vi "DiffDriveSim_Create_Model.vi"(6 "Encoder Counts/Rev":dbl=360.0, 7 "Robot Physical Info":T1={"Mass_LB"=3.0, "Actual TrackWidth Inch"=21.0, "Skid Factor"=1.75} {"Actual TrackWidth Inch" format="%#_13g"}, 8 "Use Custom Drive":bool, 9 "Custom Drive Info":T6={"Motor Type"=enum."Romi BuiltIn", "Num Motors Per Side"=1, "Wheel Diameter Inch"=7.0, "Gear Ratio"=1.0} {"Gear Ratio" format="%#_13g"; "Wheel Diameter Inch" format="%#_13g"}, 10 "KitBot Drive Info":T2, 11 "Initial Robot Position":T8={"TRANSLATION"={"X"=0.0, "Y"=0.0}, "ROTATION"={"VALUE"=0.0, "COS"=1.0, "SIN"=0.0}} {"ROTATION"."SIN" format="%13.4f"; "ROTATION"."COS" format="%13.4f"; "ROTATION"."VALUE" format="%13.4f"; "TRANSLATION"."Y" format="%14.3f"; "TRANSLATION"."X" format="%14.3f"}) -> (2 "Encoder Ft/Count":dbl, 3 "out DiffDriveTrainSim":T11 {"m_Motor"."Jr_KgM2" format="%13.5p"; "m_Motor"."L_H" format="%13.5p"; "m_Motor"."Kt_NMPerAmp" format="%13.5p"; "m_Motor"."KvINV_RadPerSecPerVolt" format="%13.5p"; "m_Motor"."R_Ohms" format="%13.5p"; "m_Motor"."FreeSpeed_RadPerSec" format="%13.5p"; "m_Motor"."FreeCurrent_Amps" format="%13.5p"; "m_Motor"."StallCurrent_Amps" format="%13.5p"; "m_Motor"."StallTorque_NM" format="%13.5p"; "m_Motor"."nominalVoltage_Volts" format="%13.5p"})   [LabVIEW 2019]
uses:
  <vilib>/Rock Robotics/WPI/ThirdParty/JAS_Junk/TrajLib/TypeDef/DIFF_DRIVE_TRAIN_SIM.ctl
  <vilib>/Rock Robotics/WPI/ThirdParty/JAS_Junk/TrajLib/TypeDef/LINEAR_SYSTEM.ctl
  <vilib>/Analysis/Matrix/Datatypes/RealMatrix.ctl
  <vilib>/Rock Robotics/WPI/ThirdParty/JAS_Junk/TrajLib/TypeDef/DCMOTOR.CTL
  <vilib>/Rock Robotics/WPI/ThirdParty/JAS_Junk/TrajLib/TypeDef/POSE2D.ctl
  <vilib>/Rock Robotics/WPI/ThirdParty/JAS_Junk/TrajLib/TypeDef/TRANSLATION2D.ctl
  <vilib>/Rock Robotics/WPI/ThirdParty/JAS_Junk/TrajLib/TypeDef/ROTATION2D.ctl
  DiffDriveSim_CustomDriveIntoType.ctl
  <vilib>/Rock Robotics/WPI/ThirdParty/JAS_Junk/TrajLib/Enum/DCMOTOR_TYPES_ENUM.ctl
  DiffDriveSim_KitBotDriveInfoType.ctl
  <vilib>/Rock Robotics/WPI/ThirdParty/JAS_Junk/TrajLib/Enum/DIFF_DRIVE_ToughBoxMini_MotorChoice_ENUM.ctl
  <vilib>/Rock Robotics/WPI/ThirdParty/JAS_Junk/TrajLib/Enum/DIFF_DRIVE_KitBot_WheelSize_ENUM.ctl
  <vilib>/Rock Robotics/WPI/ThirdParty/JAS_Junk/TrajLib/Enum/DIFF_DRIVE_ToughBoxMini_GearChoice_ENUM.ctl
  DiffDriveSim_PhysRobotInfoType.ctl
  <vilib>/Rock Robotics/WPI/ThirdParty/JAS_Junk/TrajLib/MatBuilder_Create.vi
  <vilib>/Rock Robotics/WPI/ThirdParty/JAS_Junk/TrajLib/Trajectory_Library.lvlib
  <vilib>/Analysis/Matrix/NI_Matrix.lvlib
panel:
  # "<States, 1>"
  # "<Outputs, 1>"
  # "<Inputs, 1>"
  # "<Outputs, 1>"
  # "<States,States>"
  # "<States,Inputs>"
  # "<Outputs,States>"
  # "<Outputs,Inputs>"
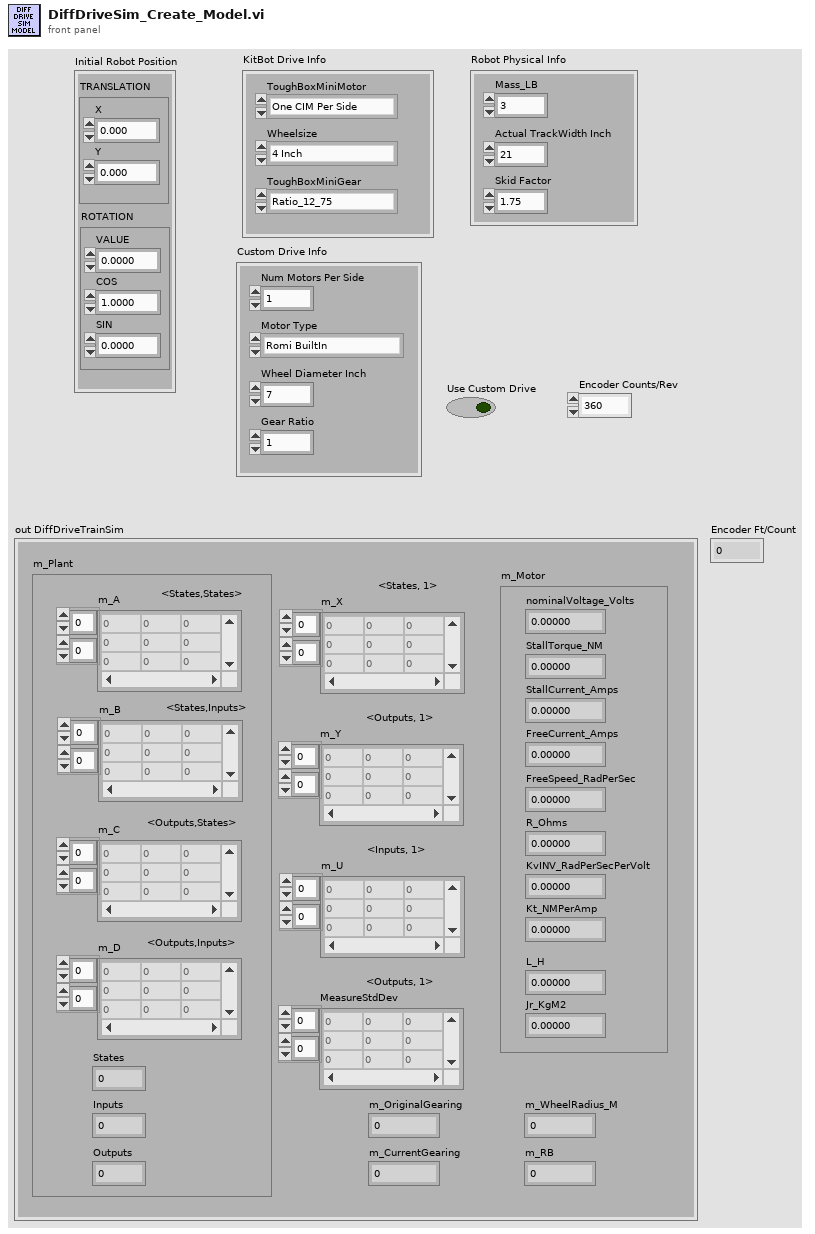
[diagram p1: front panel]
types:
  T1 = typedef "DiffDriveSim_PhysRobotInfoType.ctl" = cluster{"Mass_LB":dbl, "Actual TrackWidth Inch":dbl, "Skid Factor":dbl}
  T2 = typedef "DiffDriveSim_KitBotDriveInfoType.ctl" = cluster{"ToughBoxMiniMotor":T3, "Wheelsize":T4, "ToughBoxMiniGear":T5}
  T3 = typedef "Trajectory_Library.lvlib/DIFF_DRIVE_ToughBoxMini_MotorChoice_ENUM.ctl" = enum16{"One CIM Per Side", "Two CIM Per Side", "One MiniCIM Per Side", "Two Mini CIM Per Side", "Two Falcon Per Side", "Two NEO Per Side"}
  T4 = typedef "Trajectory_Library.lvlib/DIFF_DRIVE_KitBot_WheelSize_ENUM.ctl" = enum16{"4 Inch", "6 Inch", "8 Inch", "10 Inch"}
  T5 = typedef "Trajectory_Library.lvlib/DIFF_DRIVE_ToughBoxMini_GearChoice_ENUM.ctl" = enum16{"Ratio_12_75", "Ratio_10_71", "Ratio_8_45", "Ratio_7_31", "Ratio_5_95"}
  T6 = typedef "DiffDriveSim_CustomDriveIntoType.ctl" = cluster{"Motor Type":T7, "Num Motors Per Side":i32, "Wheel Diameter Inch":dbl, "Gear Ratio":dbl}
  T7 = typedef "Trajectory_Library.lvlib/DCMOTOR_TYPES_ENUM.ctl" = enum16{"CIM", "AndyMark 9015", "Andy Mark RS 775 125", "Bag", "BaneBots RS 550", "BaneBots RS 775", "Falcon 500", "Mini CIM", "NEO", "NEO 550", "Romi BuiltIn", "Vex 775 Pro"}
  T8 = typedef "Trajectory_Library.lvlib/POSE2D.ctl" = cluster{"TRANSLATION":T9, "ROTATION":T10}
  T9 = typedef "Trajectory_Library.lvlib/TRANSLATION2D.ctl" = cluster{"X":dbl, "Y":dbl}
  T10 = typedef "Trajectory_Library.lvlib/ROTATION2D.ctl" = cluster{"VALUE":dbl, "COS":dbl, "SIN":dbl}
  T11 = typedef "Trajectory_Library.lvlib/DIFF_DRIVE_TRAIN_SIM.ctl" = cluster{"m_Plant":T12, "m_X":T13, "m_Y":T13, "m_U":T13, "MeasureStdDev":T13, "m_Motor":T14, "m_OriginalGearing":dbl, "m_CurrentGearing":dbl, "m_WheelRadius_M":dbl, "m_RB":dbl}
  T12 = typedef "Trajectory_Library.lvlib/LINEAR_SYSTEM.ctl" = cluster{"m_A":T13, "m_B":T13, "m_C":T13, "m_D":T13, "States":i32, "Inputs":i32, "Outputs":i32}
  T13 = typedef "NI_Matrix.lvlib/RealMatrix.ctl" = dbl[][]
  T14 = typedef "Trajectory_Library.lvlib/DCMOTOR.CTL" = cluster{"nominalVoltage_Volts":dbl, "StallTorque_NM":dbl, "StallCurrent_Amps":dbl, "FreeCurrent_Amps":dbl, "FreeSpeed_RadPerSec":dbl, "R_Ohms":dbl, "KvINV_RadPerSecPerVolt":dbl, "Kt_NMPerAmp":dbl, "L_H":dbl, "Jr_KgM2":dbl}
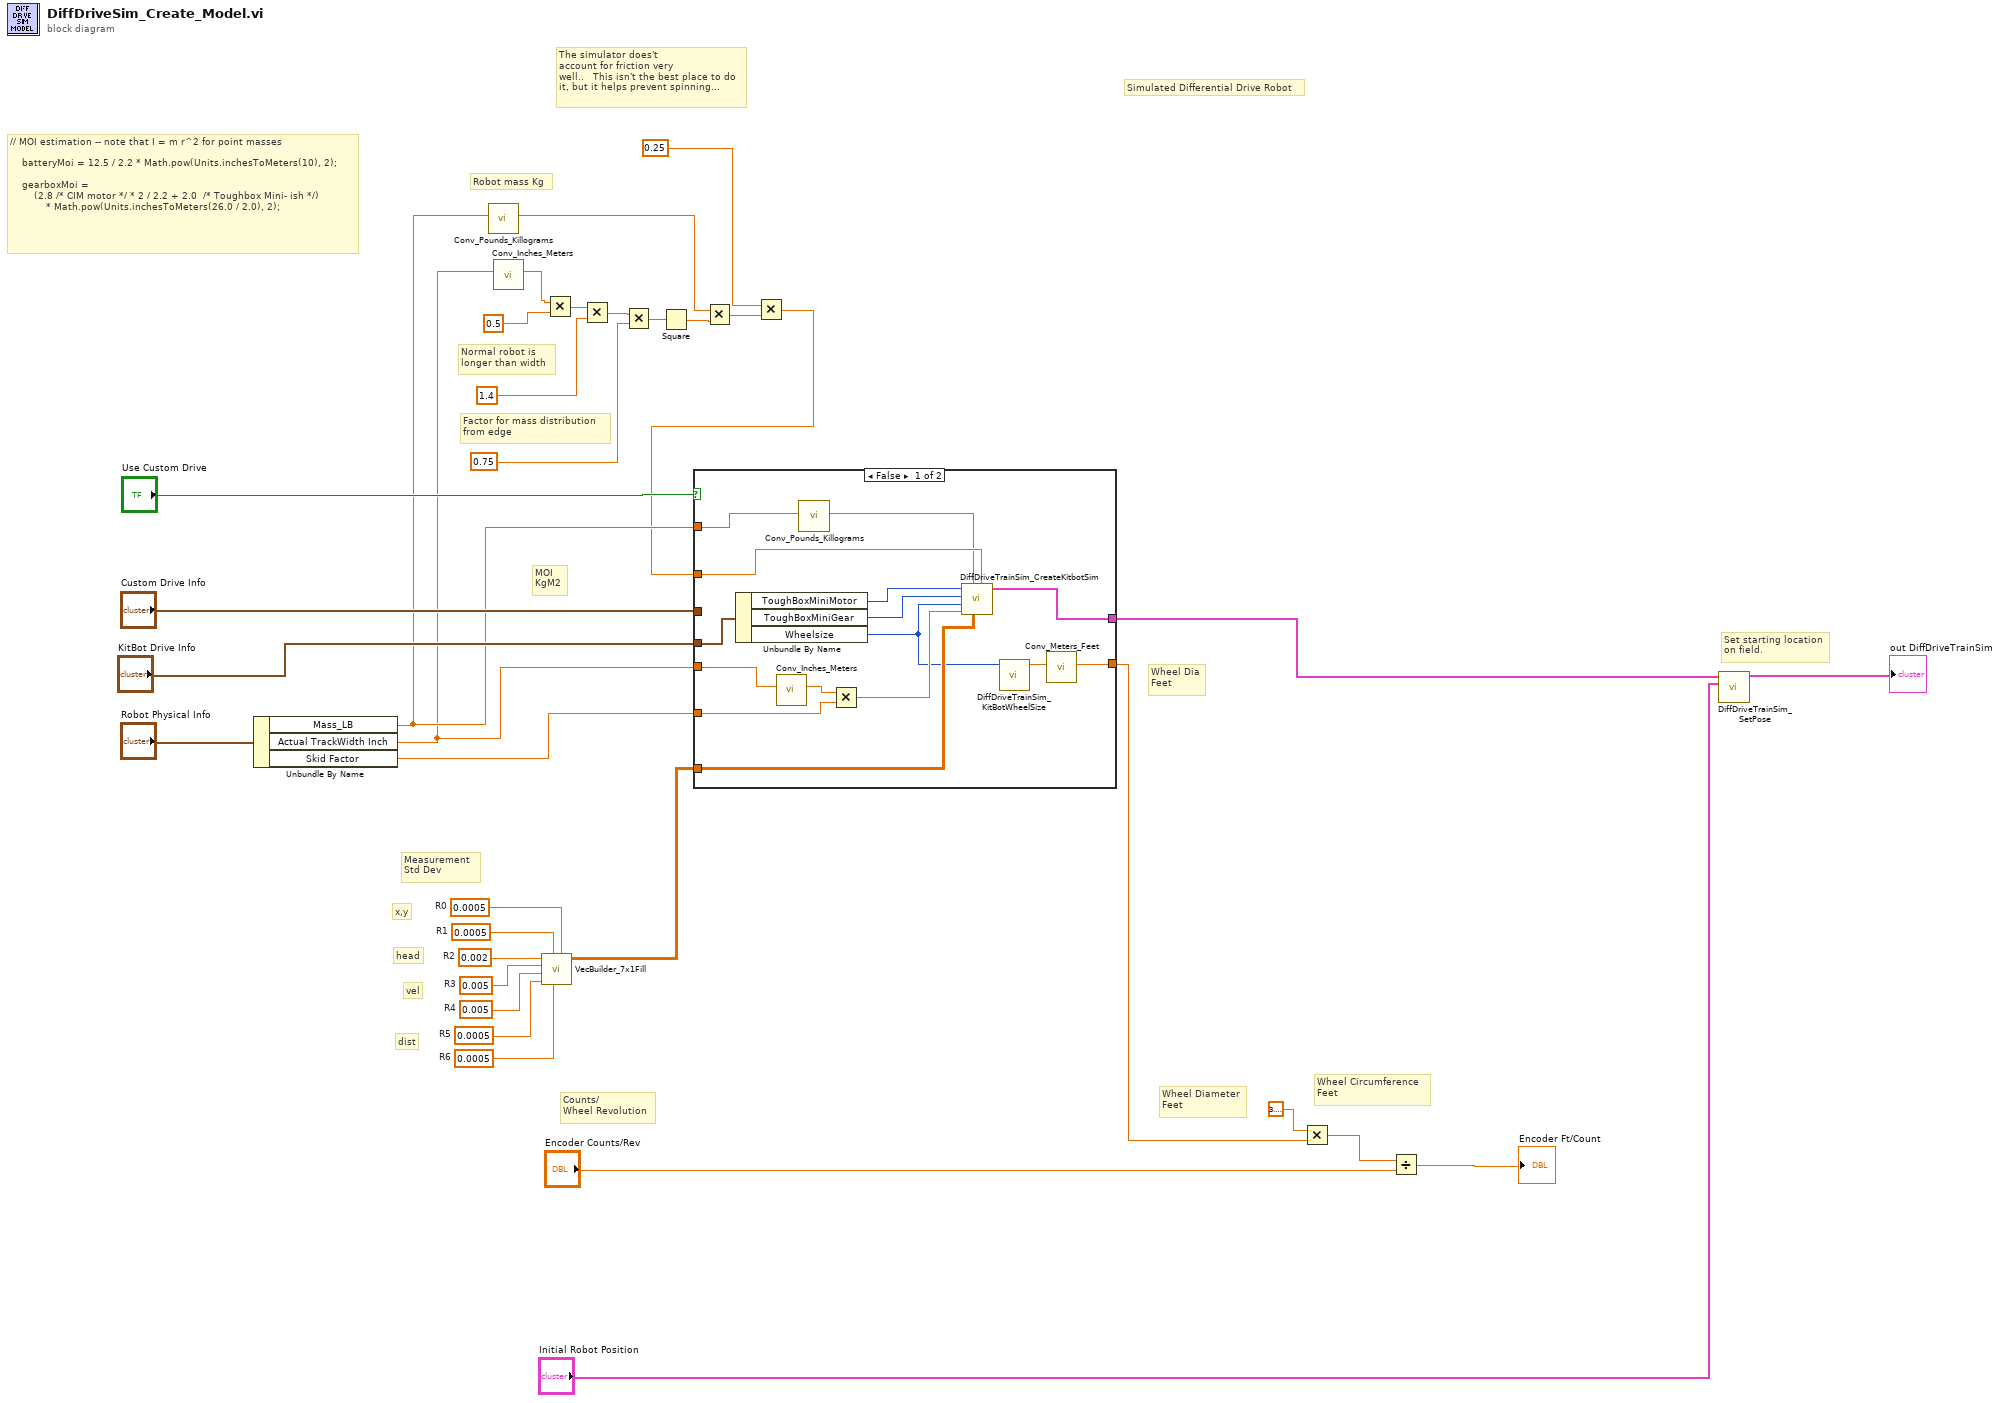
[diagram p0: block diagram]
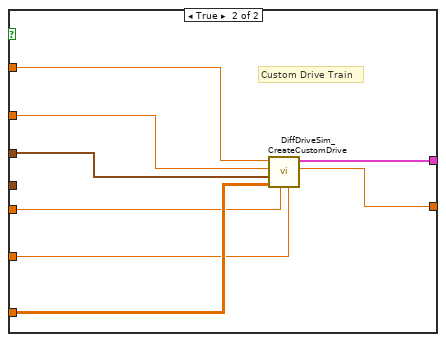
[diagram p2: hidden frame]
diagram:
  w27 = 0.0005  # R6
  w28 = 0.0005  # R5
  w29 = 0.005  # R4
  w30 = 0.005  # R3
  w31 = 0.002  # R2
  w32 = 0.0005  # R1
  w33 = 0.0005  # R0
  # "The simulator does't\naccount for friction very\nwell..   This isn't the best place to do\nit, but it helps prevent spinning..."
  # "Factor for mass distribution \nfrom edge"
  # "Normal robot is\nlonger than width"
  # "Robot mass Kg"
  # "// MOI estimation -- note that I = m r^2 for point masses\n\n    batteryMoi = 12.5 / 2.2 * Math.pow(Units.inchesToMeters(10), 2);\n\n    gearboxMoi =\n        (2.8 /* CIM motor */ * 2 / 2.2 + 2.0 \t/* Toughbox Mini- ish */)\n            * Math.pow(Units.inchesToMeters(26.0 / 2.0), 2);"
  # "Wheel Dia\nFeet"
  # "Wheel Circumference\nFeet"
  # "Wheel Diameter\nFeet"
  # "Counts/\nWheel Revolution"
  # "Set starting location\non field."
  # "Measurement \nStd Dev"
  # "MOI\nKgM2"
  # "dist"
  # "vel"
  # "head"
  # "x,y"
  # "Simulated Differential Drive Robot"
  n1 = Unbundle By Name("Robot Physical Info") -> ("Mass_LB"=w14:dbl, "Actual TrackWidth Inch"=w12:dbl, "Skid Factor"=w15:dbl)
  n2 = call <vilib>:"Conv_Pounds_Killograms.vi"("Pounds"=w14) -> ("Killograms"=w4:dbl)  [unwired: 10 in]
  n3 = call <vilib>:"Conv_Inches_Meters.vi"("INCH"=w12) -> ("Meters"=w13:dbl)  [unwired: 10 in]
  n4 = call <vilib>:"VecBuilder_7x1Fill.vi"("R0"=w33, "R6"=w27, "R1"=w32, "R5"=w28, "R4"=w29, "R3"=w30, "R2"=w31) -> ("output matrix"=w34:T13)  [unwired: 4 in]
  n5 = Multiply(x=w13, y=0.5) -> (x*y=w10:dbl)
  n6 = Multiply(x=w10, y=1.4) -> (x*y=w8:dbl)
  n7 = Multiply(x=w8, y=0.75 ("x")) -> (x*y=w6:dbl)
  n8 = Square(x=w6) -> (x^2=w5:dbl)
  n9 = Multiply(x=w4, y=w5) -> (x*y=w3:dbl)
  n10 = Multiply(x=0.25, y=w3) -> (x*y=w1:dbl)
  n11 = case shown="False" "Use Custom Drive" {
    tunnel: [w50 w58] -> w35
    tunnel: w34 -> [w39 w54]
    tunnel: w1 -> [w46 w57]
    tunnel: w14 -> [w37 w56]
    tunnel: [w48 w55] -> w18
    tunnel: "Custom Drive Info" -> [_ w53]
    tunnel: "KitBot Drive Info" -> [w47 _]
    tunnel: w12 -> [w41 w52]
    tunnel: w15 -> [w42 w51]
    frame False {
      n12 = Unbundle By Name(w47) -> ("ToughBoxMiniMotor"=w45:T3, "ToughBoxMiniGear"=w44:T5, "Wheelsize"=w38:T4)
      n13 = call <vilib>:"Conv_Inches_Meters.vi"("INCH"=w41) -> ("Meters"=w43:dbl)  [unwired: 10 in]
      n14 = call <vilib>:"Conv_Pounds_Killograms.vi"("Pounds"=w37) -> ("Killograms"=w36:dbl)  [unwired: 10 in]
      n15 = Multiply(x=w43, y=w42) -> (x*y=w40:dbl)
      n16 = call <vilib>:"DiffDriveTrainSim_CreateKitbotSim.vi"("j_KgM2"=w46, "MeasurementStdDev"=w39, "Mass_Kg"=w36, "TrackWidth_M"=w40, "Wheelsize"=w38, "ToughBoxMiniGear"=w44, "ToughBoxMiniMotor"=w45) -> ("DiffDriveTrainSim"=w50:T11)  [unwired: 3 in, 1 out]
      n17 = call <vilib>:"DiffDriveTrainSim_KitBotWheelSize.vi"("Wheel Size"=w38) -> ("WheelDiameter_M"=w49:dbl)  [unwired: 10 in]
      n18 = call <vilib>:"Conv_Meters_Feet.vi"("Meters"=w49) -> ("Feet"=w48:dbl)  [unwired: 10 in]
    }
    frame True {
      # "Custom Drive Train"
      n19 = call "DiffDriveSim_CreateCustomDrive.vi"("Skid Factor"=w51, "Actual TrackWidth Inch"=w52, "Measurement StdDev"=w54, "Custom Drive Info"=w53, "j_KgM2"=w57, "Mass_LB"=w56) -> ("Meters"=w55:dbl, "DiffDriveTrainSim"=w58:T11)  [unwired: 4 in]
    }
  }
  n20 = Multiply(x=3.141592653589793, y=w18) -> (x*y=w24:dbl)
  n21 = Divide(x=w24, y="Encoder Counts/Rev") -> (x/y=→"Encoder Ft/Count":dbl)
  n22 = call <vilib>:"DiffDriveTrainSim_SetPose.vi"("Pose"="Initial Robot Position", "in DiffDriveTrainSim"=w35) -> ("out DiffDriveTrainSim"=→"out DiffDriveTrainSim":T11)  [unwired: 9 in]
